vi "AskForCreateNewDir.vi"(11 "Experiment base path":path) -> ()   [LabVIEW 2011]
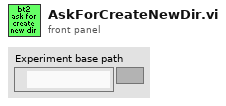
[diagram p1: front panel]
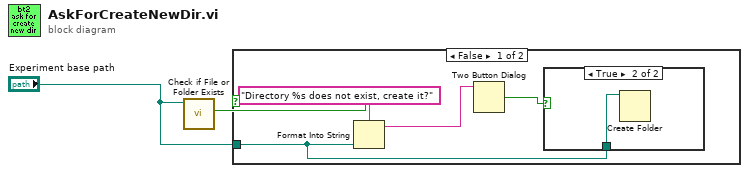
[diagram p0: block diagram]
diagram:
  n1 = call <vilib>:"Check if File or Folder Exists.vi"("path"="Experiment base path") -> ("file or folder exists?"=w2:bool)  [unwired: 8 in, 2 out]
  n2 = case shown="False" w2 {
    tunnel: "Experiment base path" -> [w3 _]
    frame False {
      n3 = Format Into String(format string="Directory %s does not exist, create it?", w3) -> (resulting string=w5:string)  [unwired: 2 in, 1 out]
      n4 = Two Button Dialog(message=w5) -> (T button?=w4:bool)  [unwired: 2 in]
      n5 = case shown="True" w4 {
        tunnel: w3 -> [_ w7]
        frame False {
        }
        frame True {
          n6 = Create Folder(path (use dialog)=w7) -> ()  [unwired: 2 in, 3 out]
        }
      }
    }
    frame True {
    }
  }
